vi "AI-usb-test all v10.vi"() -> ()   [LabVIEW 2013]
panel:
  in  "Tab Control":enum32{"Page 1", "Page 2", "Page 3"}(tab)
  in  "rate":dbl
  in  "samples":dbl
  out "TASK USB 0":i32
  out "TASK USB 1":i32
  out "TASK USB 2":i32
  out "error array":errorcluster[](array[cluster])
  out "AI Task Er":bool
  out "data 0":waveform(dbl)[](array[waveform])
  out "data 1":waveform(dbl)[](array[waveform])
  out "data 2":waveform(dbl)[](array[waveform])
  out "error array 2":errorcluster[](array[cluster])
  out "graph 2":waveform(dbl)[](graph)
  out "graph 1":waveform(dbl)[](graph)
  out "graph 0":waveform(dbl)[](graph)
  out "loop time":dbl format="%.6g"
  in  "stop":bool
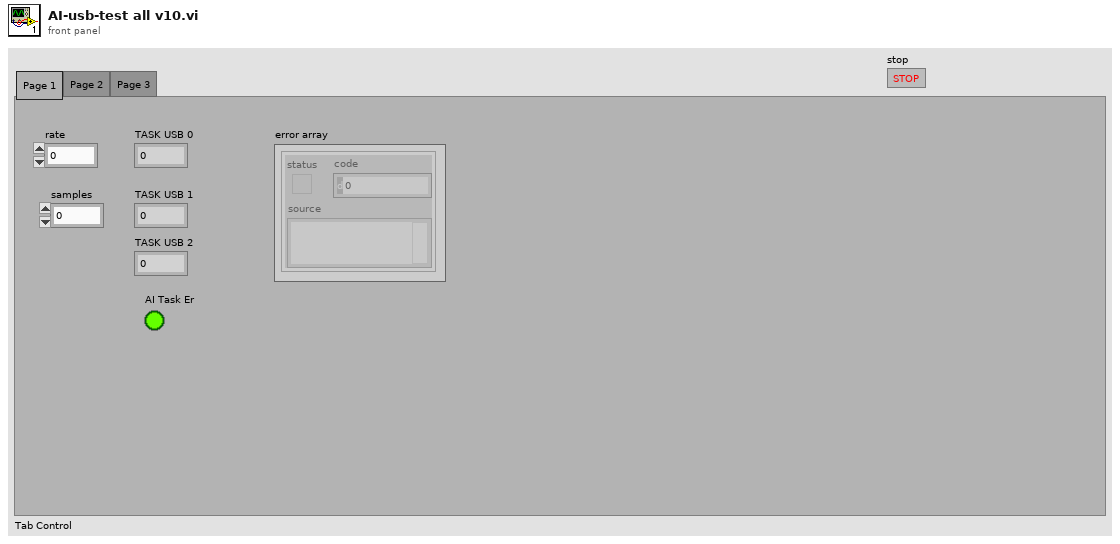
[diagram p1: front panel]
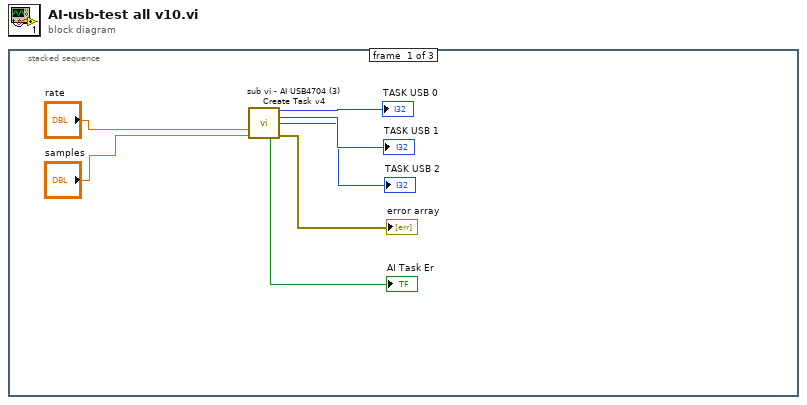
[diagram p0: block diagram]
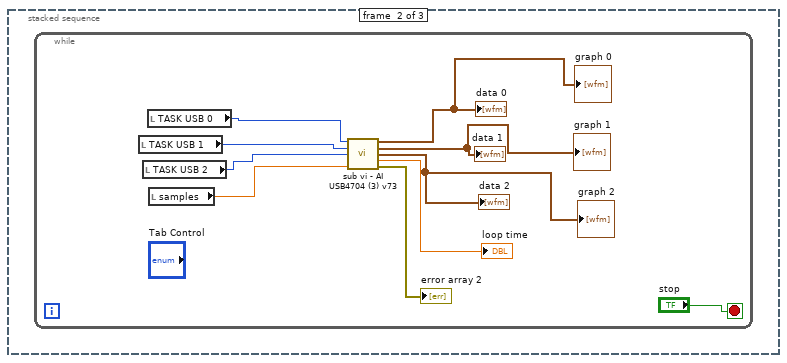
[diagram p2: hidden frame]
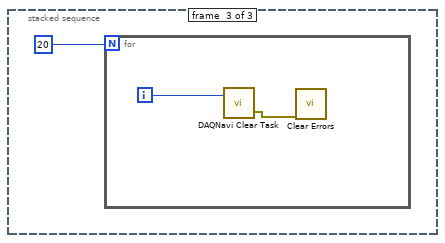
[diagram p3: hidden frame]
diagram:
  n1 = stacked-sequence {
    frame #0 {
      n2 = call "sub vi - AI USB4704 (3)  Create Task v4.vi"("Rate Hz"="rate", "Samples"="samples") -> ("TASK USB 0"=→"TASK USB 0":i32, "TASK USB 1"=→"TASK USB 1":i32, "TASK USB 2"=→"TASK USB 2":i32, "AI Task Er"=→"AI Task Er":bool, "error array"=→"error array":errorcluster[])  [unwired: 9 in]
    }
    frame #1 {
      n3 = while {
        stop <- "stop" stop-if-true
        n4 = local read "TASK USB 1"() -> (w16:i32)
        n5 = local read "TASK USB 2"() -> (w15:i32)
        n6 = local read "TASK USB 0"() -> (w17:i32)
        n7 = local read "samples"() -> (w14:dbl)
        n8 = call "sub vi - AI USB4704 (3) v73.vi"("Task0"=w17, "Task1"=w16, "Task2"=w15, "SAMPLES"=w14) -> ("data 0"=→"data 0" →"graph 0":waveform(dbl)[], "data 1"=→"data 1" →"graph 1":waveform(dbl)[], "data 2"=→"data 2" →"graph 2":waveform(dbl)[], "loop time"=→"loop time":dbl, "error array"=→"error array 2":errorcluster[])  [unwired: 7 in]
      }
    }
    frame #2 {
      n9 = for {
        N: 20 -> [_]
        i -> [w19]
        n10 = call <userlib>:"DAQNavi Clear Task.vi"("task in"=w19) -> ("error out"=w20:errorcluster)  [unwired: 2 in]
        n11 = call <vilib>:"Clear Errors.vi"("error in (no error)"=w20) -> ()  [unwired: 6 in, 1 out]
      }
    }
  }
